vi "Flatten.vi"(8 "error in":errorcluster, 9 "Data":T1) -> (0 "error out":errorcluster, 2 "Buffer":u8[](array[numeric]) format="%.0x")   [LabVIEW 2020, in "SyncTicks.lvlib"]
uses:
  SyncTicks.lvlib
  Data.ctl
  lv-protoc/LV-Proto/LV-Proto.lvlib
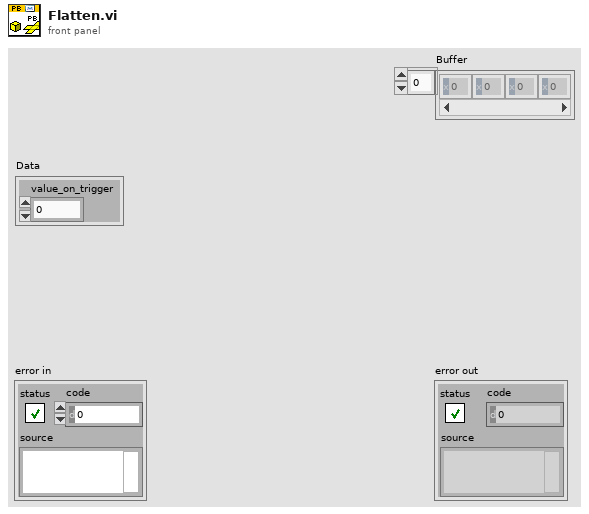
[diagram p1: front panel]
types:
  T1 = typedef "SyncTicks.lvlib/Data.ctl" = cluster{"value_on_trigger":u32}
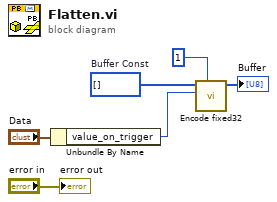
[diagram p0: block diagram]
diagram:
  w4 = u8[] []  # Buffer Const
  n1 = Unbundle By Name("Data") -> ("value_on_trigger"=w2:u32)
  n2 = call "Encode fixed32.vi"("Field Number"=1, "fixed32"=w2, "Buffer in"=w4) -> ("Buffer"=→"Buffer":u8[])  [unwired: 8 in]
  "error out" <- "error in"
